vi "CalculateUncertraintyForRealPartWhenImagisZero.vi"(9 "Extinction ExtinctionUncertainity Size parameter and Number ofS sizes 2":T1={"Extinction"=[], "Extinction Uncertainty"=[], "Size parameters"=[], "Number ofSizes"=0.0, "GeometricCrossSection"=[], "Wave Length"=0.0, "SMPS Sizes"=[], "Concentration"=[], "Double Charge Correction"=FALSE, "Extincation Factor"=1.0, "Diameter Factor"=1.0, "Diameter Offset"=0.0, "Extinction Factor Flag"=FALSE, "Diameter Factor Flag"=FALSE, "Diameter Offset Flag"=FALSE, "Sizes"=[], "ExtinctionOrAbsorptionOrScattering"=0} {"ExtinctionOrAbsorptionOrScattering" scale=0.0..2.0}, 10 "refractive index, imaginary":dbl=0.10000000149011612 step=0.001 format="%.3f", 11 "refractive index, real":dbl=1.2999999523162842 step=0.001 format="%.3f") -> (3 "Uncertainty in the Real Part":dbl=0.10000000149011612 step=0.001 format="%.3f")   [LabVIEW 2013]
uses:
  BaesDataTypeDefinition.ctl
  <vilib>/gmath/zero.llb/Newton Raphson Zero Finder (VI).vi
  <vilib>/gmath/NI_Gmath.lvlib
panel:
  in  "cluster":T2={"Imaginary or Real Part"=0.0, "Chi Square at Minimum"=0.0, "Extinction ExtinctionUncertainity Size parameter and Number ofS sizes"={"Extinction"=[], "Extinction Uncertainty"=[], "Size parameters"=[], "Number ofSizes"=0.0, "GeometricCrossSection"=[], "Wave Length"=0.0, "SMPS Sizes"=[], "Concentration"=[], "Double Charge Correction"=FALSE, "Extincation Factor"=1.0, "Diameter Factor"=1.0, "Diameter Offset"=0.0, "Extinction Factor Flag"=FALSE, "Diameter Factor Flag"=FALSE, "Diameter Offset Flag"=FALSE, "Sizes"=[], "ExtinctionOrAbsorptionOrScattering"=0}} {"Extinction ExtinctionUncertainity Size parameter and Number ofS sizes"."ExtinctionOrAbsorptionOrScattering" scale=0.0..2.0}
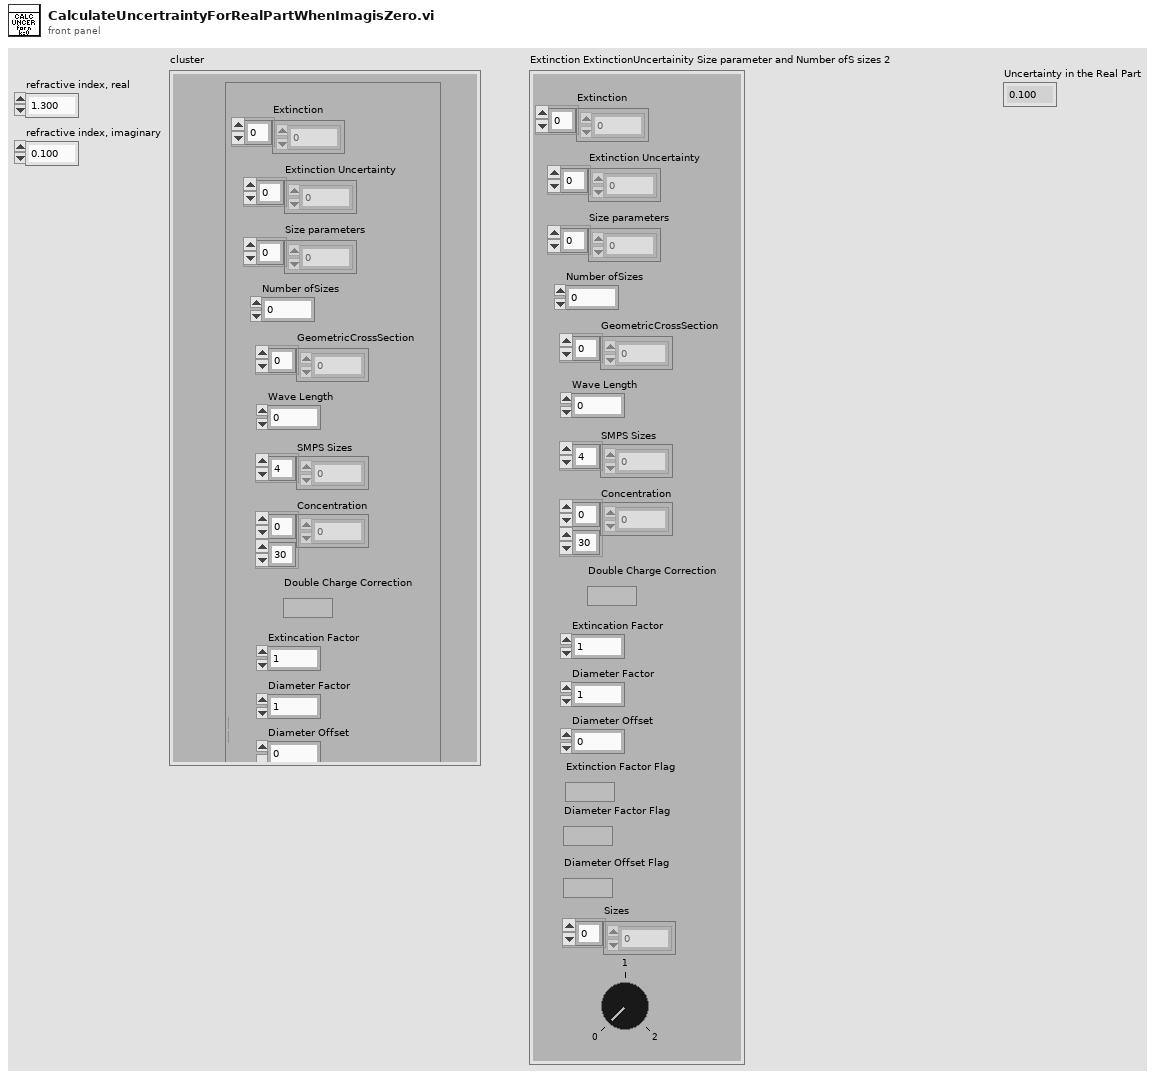
[diagram p1: front panel]
types:
  T1 = typedef "BaesDataTypeDefinition.ctl" = cluster{"Extinction":dbl[], "Extinction Uncertainty":dbl[], "Size parameters":dbl[], "Number ofSizes":dbl, "GeometricCrossSection":dbl[], "Wave Length":dbl, "SMPS Sizes":dbl[], "Concentration":dbl[][], "Double Charge Correction":bool, "Extincation Factor":dbl, "Diameter Factor":dbl, "Diameter Offset":dbl, "Extinction Factor Flag":bool, "Diameter Factor Flag":bool, "Diameter Offset Flag":bool, "Sizes":dbl[], "ExtinctionOrAbsorptionOrScattering":i8}
  T2 = cluster{"Imaginary or Real Part":dbl, "Chi Square at Minimum":dbl, "Extinction ExtinctionUncertainity Size parameter and Number ofS sizes":T1}
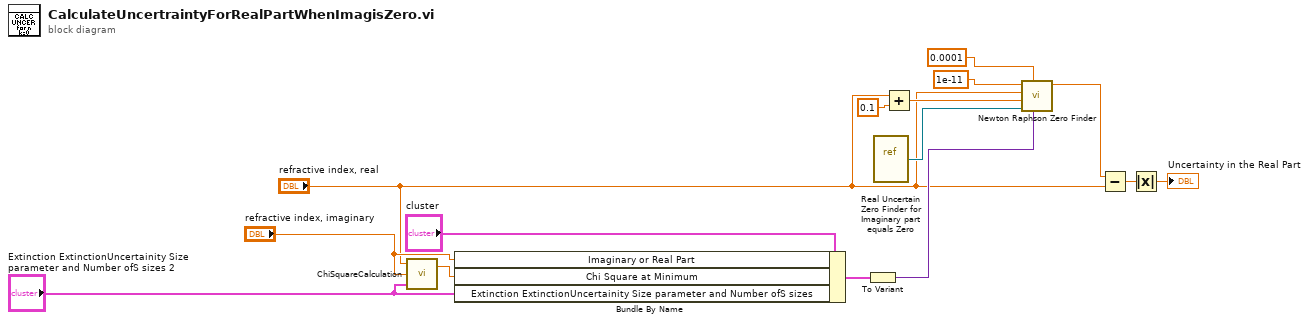
[diagram p0: block diagram]
diagram:
  n1 = call "ChiSquareCalculation.vi"("Extinction ExtinctionUncertainity Size parameter and Number ofS sizes 2"="Extinction ExtinctionUncertainity Size parameter and Number ofS sizes 2", "refractive index, imaginary"="refractive index, imaginary", "refractive index, real"="refractive index, real") -> ("Chi Squared"=w6:dbl)  [unwired: 1 out]
  n2 = Bundle By Name(cluster="cluster", "Imaginary or Real Part"="refractive index, imaginary", "Chi Square at Minimum"=w6, "Extinction ExtinctionUncertainity Size parameter and Number ofS sizes"="Extinction ExtinctionUncertainity Size parameter and Number ofS sizes 2") -> (w15:T2)
  n3 = To Variant(anything=w15) -> (Variant=w14:variant)
  n4 = vi-ref "Real Uncertain Zero Finder for Imaginary part equals Zero.vi"() -> (w11:refnum<vi>)
  n5 = Add(x="refractive index, real", y=0.1) -> (x+y=w12:dbl)
  n6 = call-poly <vilib>:"Newton Raphson Zero Finder.vi"("data"=w14, "accuracy"=0.0001, "f(x)"=w11, "end"=w12, "start"="refractive index, real", "h"=1e-11) -> ("zero"=w4:dbl)  [unwired: 2 in, 3 out]
  n7 = Subtract(x=w4, y="refractive index, real") -> (x-y=w2:dbl)
  n8 = Absolute Value(x=w2) -> (abs(x)=→"Uncertainty in the Real Part":dbl)
